vi "ASK Receiver.vi"() -> ()   [LabVIEW 2015]
uses:
  <instrlib>/niUSRP/niUSRP Fetch Rx Data (CDB WDT).vi
panel:
  out "Demodulated Signal":dbl(graph)
  out "Received Signal":dbl(graph)
  in  "y":bool
  in  "active antenna":string
  out "error out":errorcluster
  in  "number of samples":i64=1000
  out "coerced gain":dbl format="%#_6f"
  out "coerced carrier frequency":dbl=100000.0 format="%#_6p"
  out "coerced IQ rate":dbl=100000.0 format="%#_6p"
  in  "gain":dbl format="%#_6f"
  in  "carrier frequency":dbl=100000.0 format="%#_6p"
  in  "IQ rate":dbl=100000.0 format="%#_6p"
  in  "device names":refnum<k15>
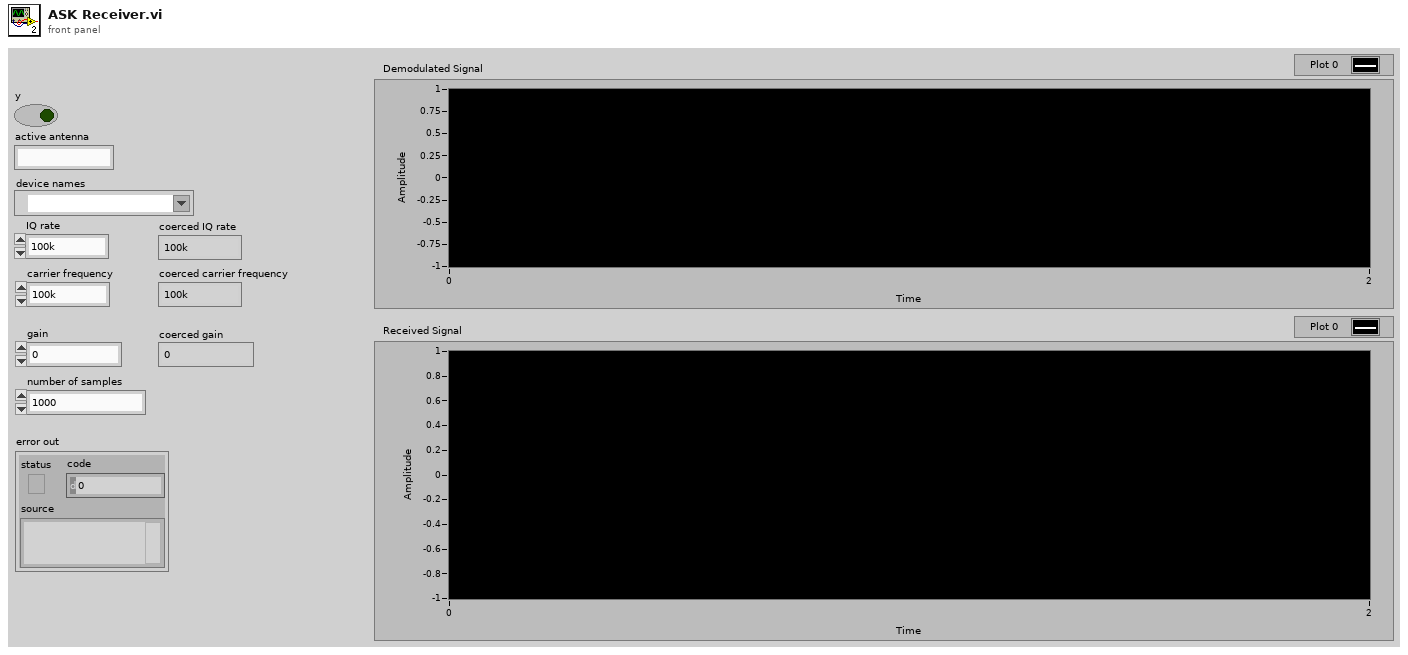
[diagram p1: front panel]
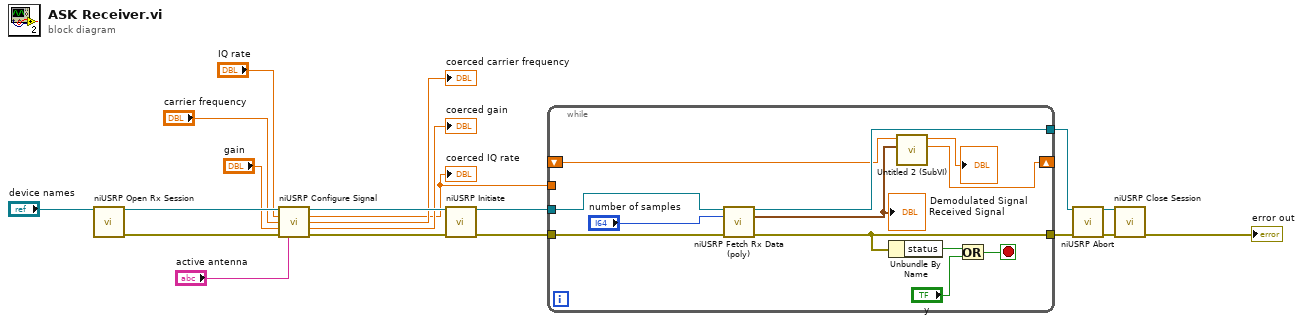
[diagram p0: block diagram]
diagram:
  n1 = call <instrlib>:"niUSRP Open Rx Session.vi"("device names"="device names") -> ("session handle out"=w19:refnum<k15>, "error out"=w18:errorcluster)  [unwired: 13 in]
  n2 = call <instrlib>:"niUSRP Configure Signal.vi"("session handle"=w19, "IQ rate"="IQ rate", "carrier frequency"="carrier frequency", "gain"="gain", "error in (no error)"=w18, "active antenna"="active antenna") -> ("session handle out"=w17:refnum<k15>, "coerced IQ rate"=w9:dbl, "coerced carrier frequency"=→"coerced carrier frequency":dbl, "coerced gain"=→"coerced gain":dbl, "error out"=w16:errorcluster)  [unwired: 5 in]
  "coerced IQ rate" <- w9
  n3 = call <instrlib>:"niUSRP Initiate.vi"("session handle"=w17, "error in (no error)"=w16) -> ("session handle out"=w3:refnum<k15>, "error out"=w4:errorcluster)  [unwired: 12 in]
  n4 = while {
    tunnel: w9 -> [_]
    tunnel: [w28] -> w5
    tunnel: [w27] -> w1
    tunnel: w4 -> [w26]
    tunnel: w3 -> [w25]
    shift-right: [w23] -> _
    shift-left: _ -> [w22]
    stop <- w24 stop-if-true
    n5 = call-poly <instrlib>:"niUSRP Fetch Rx Data (poly).vi"("session handle"=w25, "number of samples"="number of samples", "error in (no error)"=w26) -> ("session handle out"=w28:refnum<k15>, "data"=w20:waveform(cdb), "error out"=w27:errorcluster)  [unwired: 9 in, 1 out]
    "Received Signal" <- w20
    n6 = Unbundle By Name(w27) -> ("status"=w30:bool)
    n7 = call "Untitled 2 (SubVI).vi"("x"=w20, "x 2"=w22) -> ("s? t:f 3"=w23:dbl, "s? t:f"=→"Demodulated Signal":dbl)  [unwired: 8 in]
    n8 = Or(x=w30, y="y") -> (x .or. y?=w24:bool)
  }
  n9 = call <instrlib>:"niUSRP Abort.vi"("session handle"=w5, "error in (no error)"=w1) -> ("session handle out"=w8:refnum<k15>, "error out"=w7:errorcluster)  [unwired: 12 in]
  n10 = call <instrlib>:"niUSRP Close Session.vi"("session handle"=w8, "error in (no error)"=w7) -> ("error out"=→"error out":errorcluster)  [unwired: 13 in]
